vi "__List Drop Handler.vi"(7 "FileManager Data":T1, 8 "error in (no error)":errorcluster, 10 "Available data names":string[](array[string]), 11 "MCListbox Refnum":refnum<vi>) -> (0 "error out":errorcluster, 3 "Accept?":bool)   [LabVIEW 2011]
doc: "This VI is responsible for taking the necessary action when a drag and drop operation finishes.\nIf the operation is permitted, it will upload or download a file to/from the cloud."
uses:
  __File manager Data type.ctl
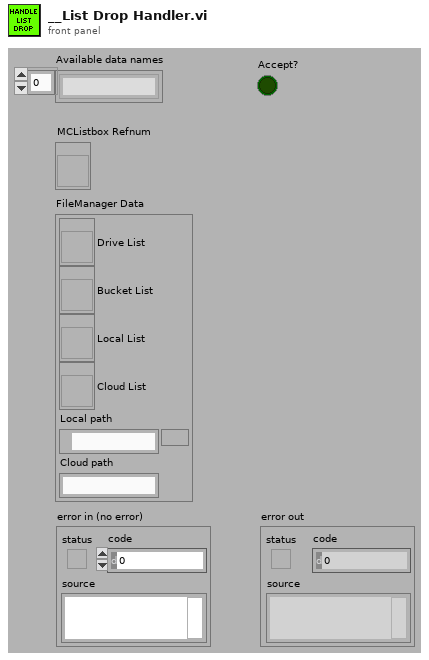
[diagram p1: front panel]
types:
  T1 = typedef "__File manager Data type.ctl" = cluster{"Drive List":refnum<vi>, "Bucket List":refnum<vi>, "Local List":refnum<vi>, "Cloud List":refnum<vi>, "Local path":path, "Cloud path":string}
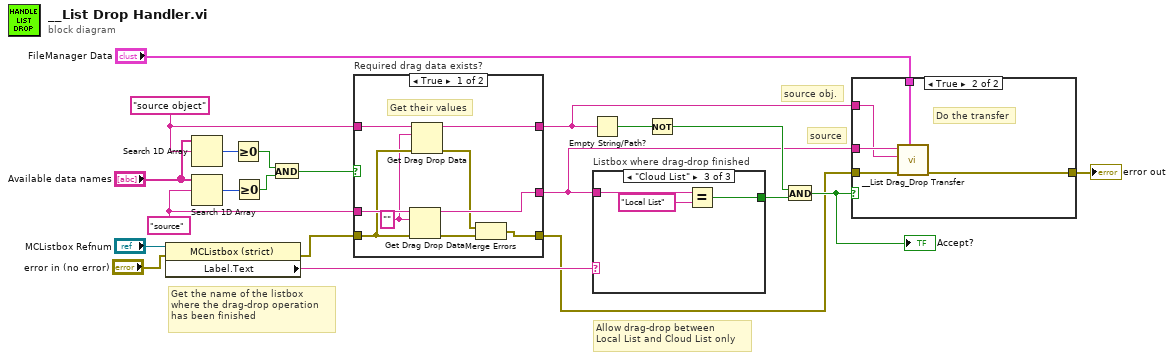
[diagram p0: block diagram]
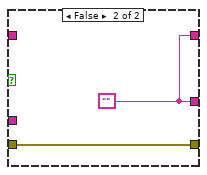
[diagram p3: hidden frame]
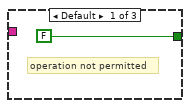
[diagram p4: hidden frame]
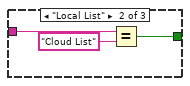
[diagram p5: hidden frame]
diagram:
  w10 = "source object"
  w18 = "source"
  # "Get the name of the listbox\nwhere the drag-drop operation\nhas been finished"
  # "Allow drag-drop between\nLocal List and Cloud List only"
  # "source"
  # "source obj."
  n1 = property class="MCListbox (strict)"(reference="MCListbox Refnum", error in="error in (no error)") -> (error out=w17:errorcluster, "Label.Text"=w19:string)  [unwired: 1 out]
  n2 = Search 1D Array(1D array="Available data names", element=w10) -> (index of element=w14:i32)  [unwired: 1 in]
  n3 = Search 1D Array(1D array="Available data names", element=w18) -> (index of element=w15:i32)  [unwired: 1 in]
  n4 = Greater Or Equal To 0?(x=w14) -> (x >= 0?=w13:bool)
  n5 = Greater Or Equal To 0?(x=w15) -> (x >= 0?=w12:bool)
  n6 = And(x=w13, y=w12) -> (x .and. y?=w11:bool)
  n7 = case "Required drag data exists?" shown="True" w11 {
    tunnel: w17 -> [w28 w32]
    tunnel: w18 -> [w30 _]
    tunnel: [w22 w32] -> w3
    tunnel: [w29 w31] -> w4
    tunnel: w10 -> [w27 _]
    tunnel: [w25 w31] -> w5
    frame True {
      w26 = "" ("type")
      # "Get their values"
      n8 = Get Drag Drop Data(6:w28, 8:w26, 9:w30) -> (0:w24:errorcluster, 3:w29:string)
      n9 = Get Drag Drop Data(6:w28, 8:w26, 9:w27) -> (0:w23:errorcluster, 3:w25:string)
      n10 = Merge Errors(w23, w24) -> (w22:errorcluster)
    }
    frame False {
      w31 = ""
    }
  }
  n11 = Empty String/Path?(string/path=w5) -> (empty?=w9:bool)
  n12 = case "Listbox where drag-drop finished" shown="\"Cloud List\"" w19 {
    tunnel: w4 -> [_ w36 w39]
    tunnel: [FALSE w34 w37] -> w8
    frame Default {
      # "operation not permitted"
    }
    frame "Local List" {
      n13 = Equal?(x=w36, y="Cloud List") -> (x = y?=w34:bool)
    }
    frame "Cloud List" {
      n14 = Equal?(x=w39, y="Local List") -> (x = y?=w37:bool)
    }
  }
  n15 = Not(x=w9) -> (.not. x?=w7:bool)
  n16 = And(x=w7, y=w8) -> (x .and. y?=w6:bool)
  "Accept?" <- w6
  n17 = case shown="True" w6 {
    tunnel: w5 -> [_ w43]
    tunnel: w4 -> [_ w45]
    tunnel: w3 -> [w40 w44]
    tunnel: "FileManager Data" -> [_ w42]
    tunnel: [w40 w41] -> w1
    frame False {
      # "unaccepted operation, do nothing"
    }
    frame True {
      # "Do the transfer"
      n18 = call "__List Drag_Drop Transfer.vi"("FileManager Data"=w42, "error in (no error)"=w44, "Source Object"=w43, "Source"=w45) -> ("error out"=w41:errorcluster)  [unwired: 7 in]
    }
  }
  "error out" <- w1
